vi "filterCreateMsg.vi"(7 "time elapsed?":bool, 8 "error in (no error)":errorcluster, 9 "auto sweep (true)":bool=TRUE, 10 "filtering (true)":bool=TRUE, 11 "queue in":refnum<queue>) -> (0 "error out":errorcluster, 3 "queue out":refnum<queue>)   [LabVIEW 2011]
uses:
  QMH/QMH Add Message to Queue (Single Element).vi
  QMH/QMH Add Message to Queue (Array).vi
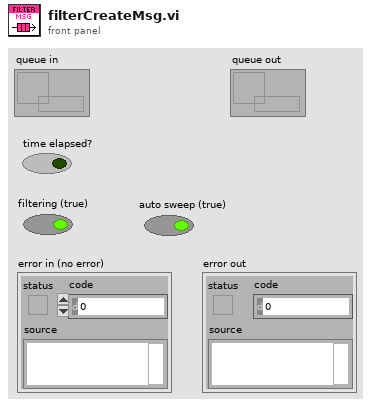
[diagram p1: front panel]
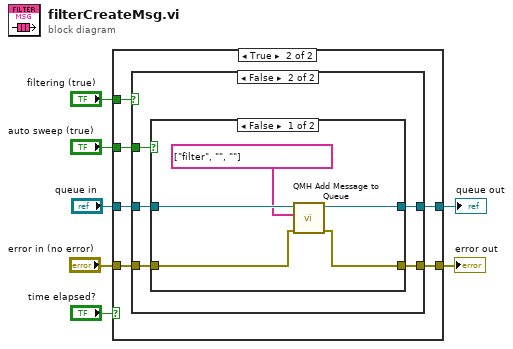
[diagram p0: block diagram]
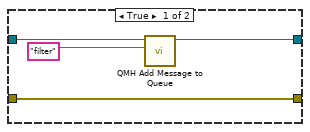
[diagram p3: hidden frame]
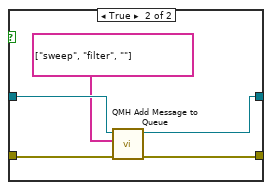
[diagram p4: hidden frame]
diagram:
  n1 = case shown="True" "time elapsed?" {
    tunnel: "queue in" -> [w8 w15]
    tunnel: "auto sweep (true)" -> [_ w14]
    tunnel: "filtering (true)" -> [_ w13]
    tunnel: [w9 w12] -> w6
    tunnel: "error in (no error)" -> [w9 w11]
    tunnel: [w8 w10] -> w1
    frame False {
    }
    frame True {
      n2 = case shown="False" w13 {
        tunnel: w15 -> [w17 w24]
        tunnel: w14 -> [_ w23]
        tunnel: [w19 w22] -> w12
        tunnel: w11 -> [w19 w21]
        tunnel: [w16 w20] -> w10
        frame True {
          n3 = call-poly "QMH Add Message to Queue.vi"("Message"="filter", "queue in"=w17) -> ("queue out"=w16:refnum<queue>)  [unwired: 8 in, 1 out]
        }
        frame False {
          n4 = case shown="False" w23 {
            tunnel: [w25 w31] -> w22
            tunnel: [w28 w30] -> w20
            tunnel: w24 -> [w29 w33]
            tunnel: w21 -> [w26 w34]
            frame False {
              n5 = call-poly "QMH Add Message to Queue.vi"("error in (no error)"=w26, "Messages"=string[] ["filter", "", ""], "queue in"=w29) -> ("error out"=w25:errorcluster, "queue out"=w28:refnum<queue>)  [unwired: 7 in]
            }
            frame True {
              n6 = call-poly "QMH Add Message to Queue.vi"("error in (no error)"=w34, "Messages"=string[] ["sweep", "filter", ""], "queue in"=w33) -> ("error out"=w31:errorcluster, "queue out"=w30:refnum<queue>)  [unwired: 7 in]
            }
          }
        }
      }
    }
  }
  "error out" <- w6
  "queue out" <- w1
